vi "Jeffress_model_v011.vi"() -> ()   [LabVIEW 2019]
panel:
  out "Index":string
  out "new picture":picture
  in  "stop":bool
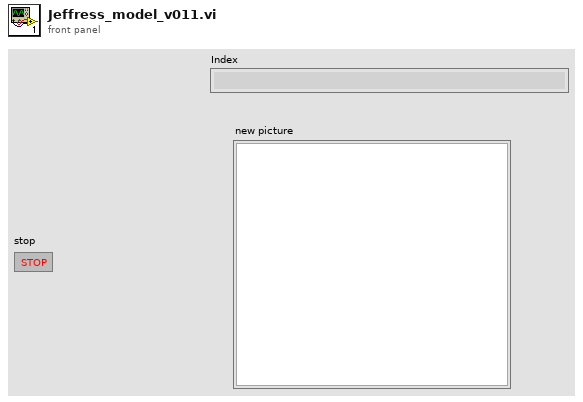
[diagram p1: front panel]
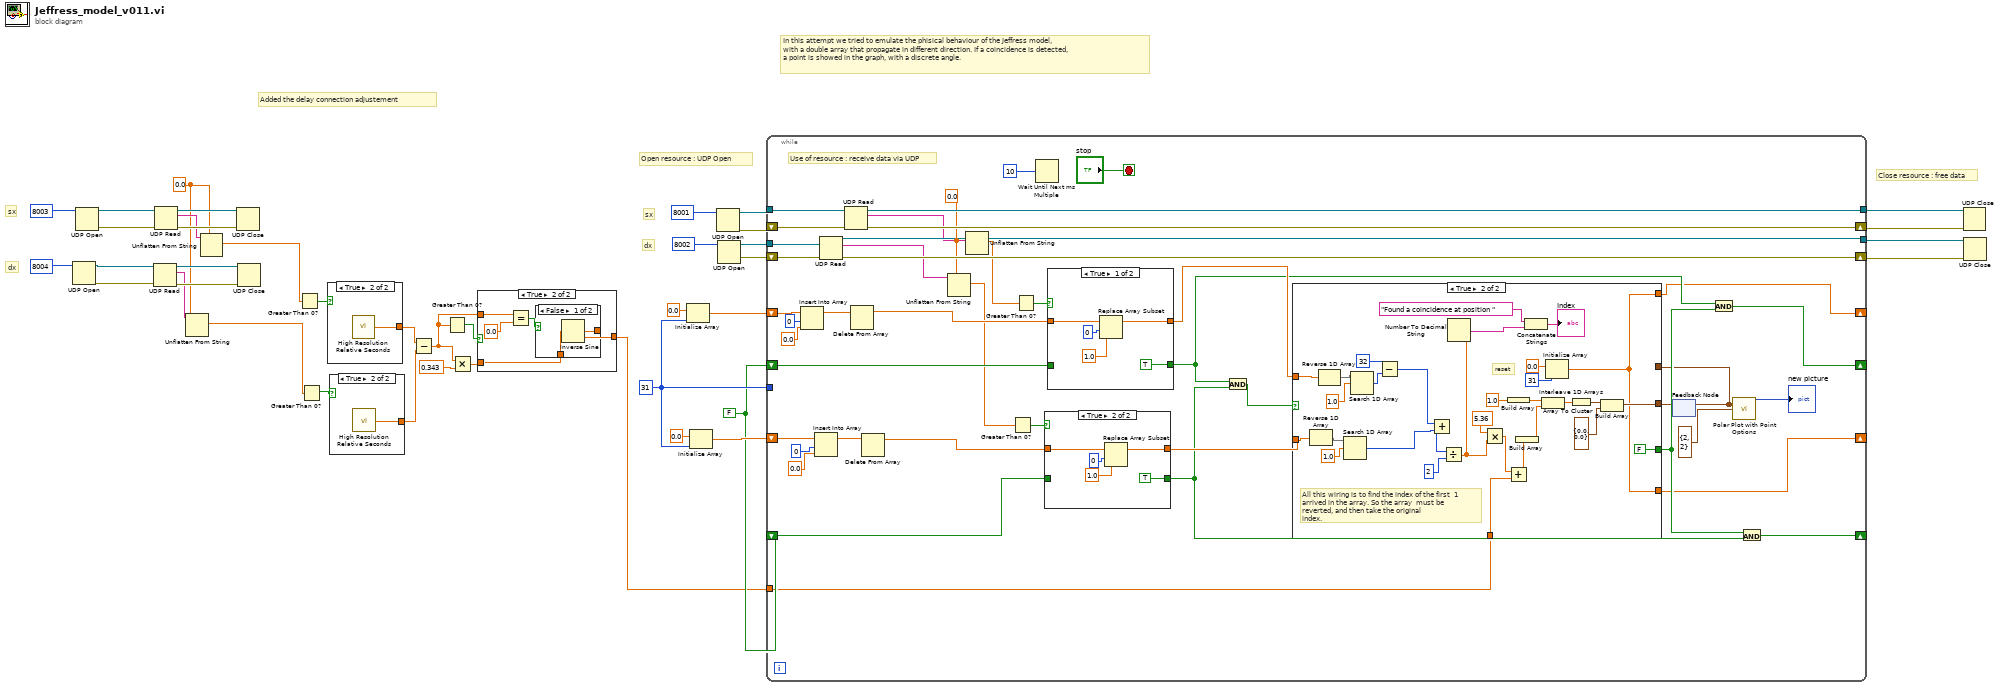
[diagram p0: block diagram]
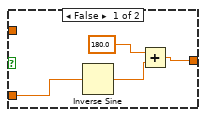
[diagram p2: hidden frame]
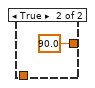
[diagram p3: hidden frame]
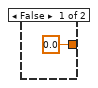
[diagram p4: hidden frame]
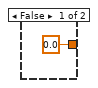
[diagram p5: hidden frame]
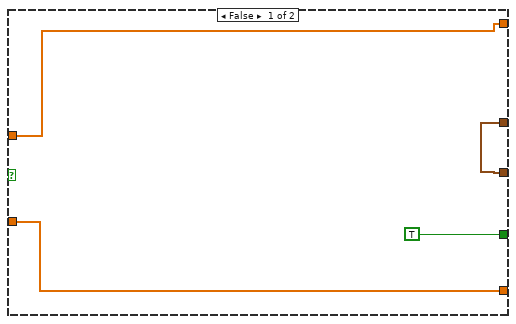
[diagram p6: hidden frame]
diagram:
  w13 = 0.0 ("element")
  w25 = FALSE
  w26 = 31 ("dimension size")
  # "dx"
  # "sx"
  # "dx"
  # "sx"
  # "Added the delay connection adjustement"
  # "In this attempt we tried to emulate the phisical behaviour of the Jeffress model,\nwith a double array that propagate in different direction. If a coincidence is detected,\na point is showed in the graph, with a discrete angle."
  # "Close resource : free data"
  # "Open resource : UDP Open"
  n1 = UDP Open(11:u16 8004) -> (port=w20:refnum<k16>, 0:w19:errorcluster)  [unwired: 4 in, 1 out]
  n2 = UDP Open(11:u16 8003) -> (port=w22:refnum<k16>, 0:w21:errorcluster)  [unwired: 4 in, 1 out]
  n3 = UDP Read(connection ID=w20, 8:w19) -> (data out=w12:string, error out=w15:errorcluster, 3:w16:refnum<k16>)  [unwired: 2 in, 2 out]
  n4 = UDP Read(connection ID=w22, 8:w21) -> (data out=w14:string, error out=w17:errorcluster, 3:w18:refnum<k16>)  [unwired: 2 in, 2 out]
  n5 = Unflatten From String(type=w13, binary string=w12) -> (value=w6:dbl)  [unwired: 3 in, 2 out]
  n6 = Unflatten From String(type=w13, binary string=w14) -> (value=w7:dbl)  [unwired: 3 in, 2 out]
  n7 = UDP Close(connection ID=w18, 8:w17) -> ()  [unwired: 2 out]
  n8 = UDP Close(connection ID=w16, 8:w15) -> ()  [unwired: 2 out]
  n9 = Greater Than 0?(x=w7) -> (x > 0?=w11:bool)
  n10 = Greater Than 0?(x=w6) -> (x > 0?=w10:bool)
  n11 = case shown="True" w11 {
    tunnel: [0.0 ("relative seconds") w42] -> w9
    frame False {
    }
    frame True {
      n12 = call <vilib>:"High Resolution Relative Seconds.vi"() -> ("relative seconds"=w42:dbl)
    }
  }
  n13 = case shown="True" w10 {
    tunnel: [0.0 ("relative seconds") w44] -> w8
    frame False {
    }
    frame True {
      n14 = call <vilib>:"High Resolution Relative Seconds.vi"() -> ("relative seconds"=w44:dbl)
    }
  }
  n15 = Subtract(x=w9, y=w8) -> (x-y=w1:dbl)
  n16 = Greater Than 0?(x=w1) -> (x > 0?=w3:bool)
  n17 = Multiply(x=w1, y=0.343) -> (x*y=w5:dbl)
  n18 = case shown="True" w3 {
    tunnel: w5 -> [w48 w52]
    tunnel: [w47 w53] -> w2
    tunnel: w1 -> [_ w49]
    frame False {
      n19 = Inverse Sine(1:w48) -> (0:w46:dbl)
      n20 = Add(x=180.0, y=w46) -> (x+y=w47:dbl)
    }
    frame True {
      n21 = Equal?(x=w49, y=0.0 ("x")) -> (x = y?=w51:bool)
      n22 = case shown="False" w51 {
        tunnel: [w55 90.0] -> w53
        tunnel: w52 -> [w54 _]
        frame False {
          n23 = Inverse Sine(1:w54) -> (0:w55:dbl)
        }
        frame True {
        }
      }
    }
  }
  n24 = Initialize Array(0.0 ("element"), w26) -> (w29:dbl[])
  n25 = Initialize Array(0.0 ("element"), w26) -> (w27:dbl[])
  n26 = UDP Open(11:u16 8001) -> (port=w38:refnum<k16>, 0:w40:errorcluster)  [unwired: 4 in, 1 out]
  n27 = UDP Open(11:u16 8002) -> (port=w34:refnum<k16>, 0:w33:errorcluster)  [unwired: 4 in, 1 out]
  n28 = while {
    tunnel: w38 -> [w96]
    tunnel: [w95] -> w37
    shift-right: [w98] -> w39
    shift-left: w40 -> [w97]
    tunnel: w34 -> [w93]
    shift-right: [w90] -> w32
    shift-left: w33 -> [w92]
    tunnel: [w91] -> w31
    shift-right: [w69] -> _
    shift-left: w29 -> [w89]
    shift-right: [w68] -> _
    shift-left: w27 -> [w81]
    tunnel: w26 -> [_]
    shift-right: [w71] -> _
    shift-left: w25 -> [w76]
    shift-right: [w70] -> _
    shift-left: w25 -> [w75]
    tunnel: w2 -> [w58]
    stop <- "stop" stop-if-true
    w63 = 0.0
    # "Use of resource : receive data via UDP"
    n29 = Insert Into Array(array=w89, index=0, new element=0.0 ("new element/subarray")) -> (w86:dbl[])
    n30 = Insert Into Array(array=w81, index=0, new element=0.0 ("new element/subarray")) -> (w82:dbl[])
    n31 = UDP Read(connection ID=w93, 8:w92) -> (data out=w64:string, error out=w90:errorcluster, 3:w91:refnum<k16>)  [unwired: 2 in, 2 out]
    n32 = UDP Read(connection ID=w96, 8:w97) -> (data out=w65:string, error out=w98:errorcluster, 3:w95:refnum<k16>)  [unwired: 2 in, 2 out]
    n33 = Delete From Array(array=w86) -> (array with subset deleted=w85:dbl[])  [unwired: 2 in, 1 out]
    n34 = Delete From Array(array=w82) -> (array with subset deleted=w80:dbl[])  [unwired: 2 in, 1 out]
    n35 = Unflatten From String(type=w63, binary string=w64) -> (value=w60:dbl)  [unwired: 3 in, 2 out]
    n36 = Unflatten From String(type=w63, binary string=w65) -> (value=w61:dbl)  [unwired: 3 in, 2 out]
    n37 = Greater Than 0?(x=w60) -> (x > 0?=w59:bool)
    n38 = Greater Than 0?(x=w61) -> (x > 0?=w62:bool)
    n39 = Wait Until Next ms Multiple(millisecond multiple=u32 10) -> ()  [unwired: 1 out]
    n40 = case shown="True" w59 {
      tunnel: [w137 w140] -> w77
      tunnel: w80 -> [w137 w139]
      tunnel: [w136 TRUE] -> w74
      tunnel: w75 -> [w136 _]
      frame False {
      }
      frame True {
        n41 = Replace Array Subset(array=w139, new element=1.0 ("new element/subarray"), index=0) -> (w140:dbl[])
      }
    }
    n42 = case shown="True" w62 {
      tunnel: [w145 w149] -> w78
      tunnel: w85 -> [w144 w149]
      tunnel: [TRUE w148] -> w72
      tunnel: w76 -> [_ w148]
      frame True {
        n43 = Replace Array Subset(array=w144, new element=1.0 ("new element/subarray"), index=0) -> (w145:dbl[])
      }
      frame False {
      }
    }
    n44 = And(x=w72, y=w74) -> (x .and. y?=w79:bool)
    n45 = feedback #1() -> (w66:cluster{"[0]":dbl, "[1]":dbl}[])  [unwired: 1 in]
    n46 = case shown="True" w79 {
      tunnel: [w101 w117] -> w67
      tunnel: w78 -> [w103 w128]
      tunnel: w77 -> [w102 w111]
      tunnel: [TRUE FALSE] -> w73
      tunnel: [w103 w113] -> w69
      tunnel: [w102 w113] -> w68
      tunnel: w66 -> [w101 _]
      tunnel: w58 -> [_ w107]
      frame False {
      }
      frame True {
        # "reset"
        # "All this wiring is to find the index of the first  1 arrived in the array. So the array  must be reverted, and then take the original \nindex."
        n47 = Reverse 1D Array(array=w111) -> (reversed array=w112:dbl[])
        n48 = Reverse 1D Array(array=w128) -> (reversed array=w127:dbl[])
        n49 = Search 1D Array(1D array=w112, element=1.0) -> (index of element=w109:i32)  [unwired: 1 in]
        n50 = Search 1D Array(1D array=w127, element=1.0) -> (index of element=w123:i32)  [unwired: 1 in]
        n51 = Subtract(x=32, y=w123) -> (x-y=w108:i32)
        n52 = Add(x=w108, y=w109) -> (x+y=w131:i32)
        n53 = Divide(x=w131, y=2) -> (x/y=w129:dbl)
        n54 = Number To Decimal String(number=w129) -> (decimal integer string=w135:string)  [unwired: 1 in]
        n55 = Multiply(x=5.36, y=w129) -> (x*y=w106:dbl)
        n56 = Build Array(1.0) -> (w121:dbl[])
        n57 = Add(x=w106, y=w107) -> (x+y=w105:dbl)
        n58 = Build Array(w105) -> (w120:dbl[])
        n59 = Concatenate Strings("Found a coincidence at position ", w135) -> (→"Index":string)
        n60 = Interleave 1D Arrays(w121, w120) -> (w119:dbl[])
        n61 = Initialize Array(0.0 ("element"), 31 ("dimension size")) -> (w113:dbl[])
        n62 = Array To Cluster(array=w119) -> (cluster=w118:cluster{"[0]":dbl, "[1]":dbl})
        n63 = Build Array(w118, cluster{"[0]":dbl, "[1]":dbl} {"[0]"=0.0, "[1]"=0.0} ("element")) -> (w117:cluster{"[0]":dbl, "[1]":dbl}[])
      }
    }
    n64 = feedback-in #1(w67) -> ()
    n65 = And(x=w72, y=w73) -> (x .and. y?=w71:bool)
    n66 = call <vilib>:"Polar Plot with Point Options.vi"("data array [mag, phase (deg)]"=w66, "top left point(0, 0)"=cluster{"x":i16, "y":i16} {"x"=2, "y"=2}) -> ("new picture"=→"new picture":picture)  [unwired: 13 in]
    n67 = And(x=w73, y=w74) -> (x .and. y?=w70:bool)
  }
  n68 = UDP Close(connection ID=w37, 8:w39) -> ()  [unwired: 2 out]
  n69 = UDP Close(connection ID=w31, 8:w32) -> ()  [unwired: 2 out]
